vi "CmdControl.vi"() -> (1 "Dataout":u8[](array[numeric]))   [LabVIEW 2017]
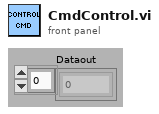
[diagram p1: front panel]
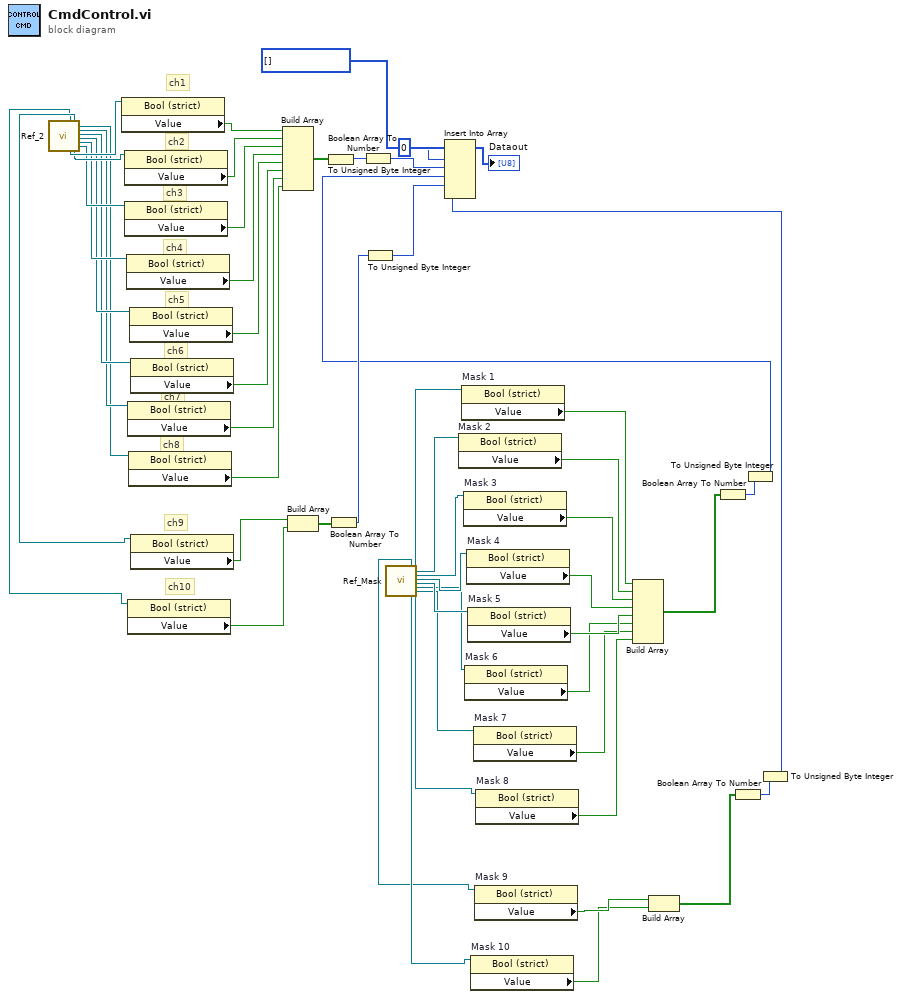
[diagram p0: block diagram]
diagram:
  # "ch10"
  # "ch9"
  # "ch8"
  # "ch7"
  # "ch6"
  # "ch5"
  # "ch4"
  # "ch3"
  # "ch2"
  # "ch1"
  n1 = call "Ref_2.vi"() -> ("Control  Ch 10 out"=w32:refnum<vi>, "Control  Ch 1 out"=w53:refnum<vi>, "Control  Ch 9 out"=w33:refnum<vi>, "Control  Ch 2 out"=w52:refnum<vi>, "Control  Ch 8 out"=w46:refnum<vi>, "Control  Ch 7 out"=w47:refnum<vi>, "Control  Ch 6 out"=w48:refnum<vi>, "Control  Ch 5 out"=w49:refnum<vi>, "Control  Ch 4 out"=w50:refnum<vi>, "Control  Ch 3 out"=w51:refnum<vi>)  [unwired: 17 in, 1 out]
  n2 = property class="Bool (strict)"(reference=w53) -> ("Value"=w45:bool)  [unwired: 1 in, 2 out]
  n3 = property class="Bool (strict)"(reference=w52) -> ("Value"=w44:bool)  [unwired: 1 in, 2 out]
  n4 = property class="Bool (strict)"(reference=w51) -> ("Value"=w43:bool)  [unwired: 1 in, 2 out]
  n5 = property class="Bool (strict)"(reference=w50) -> ("Value"=w42:bool)  [unwired: 1 in, 2 out]
  n6 = property class="Bool (strict)"(reference=w47) -> ("Value"=w39:bool)  [unwired: 1 in, 2 out]
  n7 = property class="Bool (strict)"(reference=w32) -> ("Value"=w30:bool)  [unwired: 1 in, 2 out]
  n8 = property class="Bool (strict)"(reference=w46) -> ("Value"=w38:bool)  [unwired: 1 in, 2 out]
  n9 = property class="Bool (strict)"(reference=w49) -> ("Value"=w41:bool)  [unwired: 1 in, 2 out]
  n10 = property class="Bool (strict)"(reference=w48) -> ("Value"=w40:bool)  [unwired: 1 in, 2 out]
  n11 = property class="Bool (strict)"(reference=w33) -> ("Value"=w31:bool)  [unwired: 1 in, 2 out]
  n12 = Build Array(w45, w44, w43, w42, w41, w40, w39, w38) -> (w37:bool[])
  n13 = Build Array(w31, w30) -> (w29:bool[])
  n14 = Boolean Array To Number(Boolean array=w37) -> (number=w36:u32)
  n15 = Boolean Array To Number(Boolean array=w29) -> (number=w28:u32)
  n16 = To Unsigned Byte Integer(number=w36) -> (unsigned 8bit integer=w35:u8)
  n17 = To Unsigned Byte Integer(number=w28) -> (unsigned 8bit integer=w27:u8)
  n18 = call "Ref_Mask.vi"() -> ("Mask Ch 9 out"=w7:refnum<vi>, "Mask Ch 10 out"=w8:refnum<vi>, "Mask Ch 1 out"=w16:refnum<vi>, "Mask Ch 2 out"=w15:refnum<vi>, "Mask Ch 3 out"=w14:refnum<vi>, "Mask Ch 4 out"=w13:refnum<vi>, "Mask Ch 5 out"=w12:refnum<vi>, "Mask Ch 6 out"=w11:refnum<vi>, "Mask Ch 7 out"=w10:refnum<vi>, "Mask Ch 8 out"=w9:refnum<vi>)  [unwired: 18 in]
  n19 = property on="Mask 2" class="Bool (strict)"(reference=w15) -> ("Value"=w23:bool)  [unwired: 1 in, 2 out]
  n20 = property on="Mask 1" class="Bool (strict)"(reference=w16) -> ("Value"=w24:bool)  [unwired: 1 in, 2 out]
  n21 = property on="Mask 3" class="Bool (strict)"(reference=w14) -> ("Value"=w22:bool)  [unwired: 1 in, 2 out]
  n22 = property on="Mask 6" class="Bool (strict)"(reference=w11) -> ("Value"=w19:bool)  [unwired: 1 in, 2 out]
  n23 = property on="Mask 4" class="Bool (strict)"(reference=w13) -> ("Value"=w21:bool)  [unwired: 1 in, 2 out]
  n24 = property on="Mask 5" class="Bool (strict)"(reference=w12) -> ("Value"=w20:bool)  [unwired: 1 in, 2 out]
  n25 = property on="Mask 10" class="Bool (strict)"(reference=w8) -> ("Value"=w3:bool)  [unwired: 1 in, 2 out]
  n26 = property on="Mask 7" class="Bool (strict)"(reference=w10) -> ("Value"=w18:bool)  [unwired: 1 in, 2 out]
  n27 = property on="Mask 9" class="Bool (strict)"(reference=w7) -> ("Value"=w4:bool)  [unwired: 1 in, 2 out]
  n28 = property on="Mask 8" class="Bool (strict)"(reference=w9) -> ("Value"=w17:bool)  [unwired: 1 in, 2 out]
  n29 = Build Array(w24, w23, w22, w21, w20, w19, w18, w17) -> (w25:bool[])
  n30 = Build Array(w4, w3) -> (w5:bool[])
  n31 = Boolean Array To Number(Boolean array=w25) -> (number=w26:u32)
  n32 = Boolean Array To Number(Boolean array=w5) -> (number=w6:u32)
  n33 = To Unsigned Byte Integer(number=w26) -> (unsigned 8bit integer=w2:u8)
  n34 = To Unsigned Byte Integer(number=w6) -> (unsigned 8bit integer=w1:u8)
  n35 = Insert Into Array(array=u8[] [] ("Data 2"), index=0, new element #1=w35, new element #2=w2, new element #3=w27, new element #4=w1) -> (→"Dataout":u8[])
